vi "PSA Poll OPC.vi"(8 "error in (no error)":errorcluster, 9 "Maximum Time (10000ms)":i32=10000, 11 "VISA resource name":refnum<visa-resource-name>) -> (0 "error out":errorcluster, 2 "OPC Complete?":bool, 3 "VISA resource name out":refnum<visa-resource-name>)   [LabVIEW 2014]
doc: "Waits for the current operation to finish. This VI should be called after Initiate VI.\n\n<B>Note:</B> \n\nUse this VI only with other low-level VIs. The high-level VIs automatically incorporate this functionality. This VI does not check the instrument status."
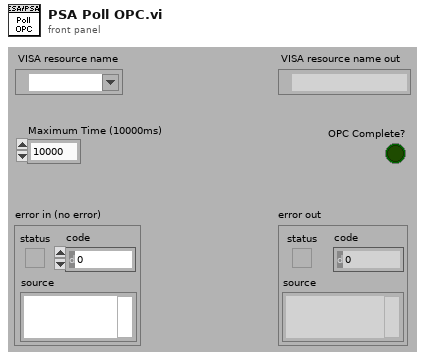
[diagram p1: front panel]
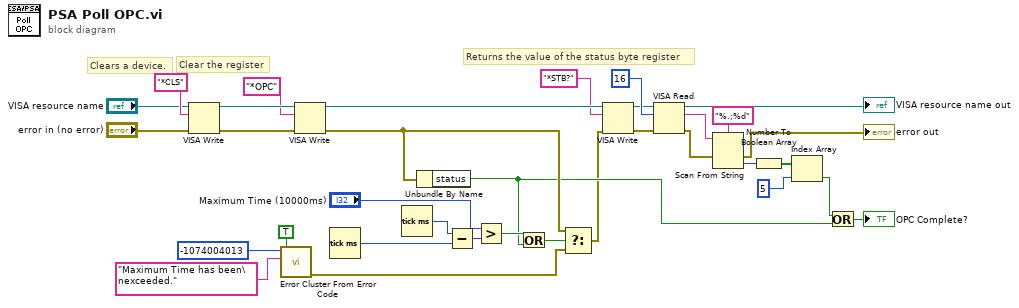
[diagram p0: block diagram]
diagram:
  # "Returns the value of the status byte register"
  # "Clears a device."
  # "Clear the register"
  n1 = VISA Write(VISA resource name="VISA resource name", write buffer="*CLS", error in (no error)="error in (no error)") -> (VISA resource name out=w24:refnum<visa-resource-name>, error out=w25:errorcluster)  [unwired: 1 out]
  n2 = call "Error Cluster From Error Code.vi"("show call chain? (False)"=TRUE, "error message (\"\")"="Maximum Time has been\nexceeded." ("error message (\"\")"), "error code (0)"=-1074004013) -> ("error out"=w28:errorcluster)  [unwired: 6 in]
  n3 = VISA Write(VISA resource name=w24, write buffer="*OPC", error in (no error)=w25) -> (VISA resource name out=w23:refnum<visa-resource-name>, error out=w22:errorcluster)  [unwired: 1 out]
  n4 = Tick Count (ms)() -> (millisecond timer value=w33:u32)
  n5 = Tick Count (ms)() -> (millisecond timer value=w12:u32)
  n6 = Unbundle By Name(w22) -> ("status"=w3:bool)
  n7 = Subtract(x=w12, y=w33) -> (x-y=w6:u32)
  n8 = Greater?(x="Maximum Time (10000ms)", y=w6) -> (0:w5:bool)
  n9 = Or(x=w5, y=w3) -> (x .or. y?=w4:bool)
  n10 = Select(t=w22, s=w4, f=w28) -> (s? t:f=w2:errorcluster)
  n11 = VISA Write(VISA resource name=w23, write buffer="*STB?", error in (no error)=w2) -> (VISA resource name out=w13:refnum<visa-resource-name>, error out=w14:errorcluster)  [unwired: 1 out]
  n12 = VISA Read(VISA resource name=w13, byte count=u32 16, error in (no error)=w14) -> (VISA resource name out=→"VISA resource name out":refnum<visa-resource-name>, read buffer=w18:string, error out=w11:errorcluster)  [unwired: 1 out]
  n13 = Scan From String(format string="%.;%d", input string=w18, error in=w11) -> (error out=→"error out":errorcluster, output 1=w8:i32)  [unwired: 2 in, 2 out]
  n14 = Number To Boolean Array(number=w8) -> (Boolean array=w9:bool[])
  n15 = Index Array(array=w9, index=5) -> (element=w7:bool)
  n16 = Or(x=w7, y=w3) -> (x .or. y?=→"OPC Complete?":bool)
